vi "Bulk Example.vi"() -> ()   [LabVIEW 2010]
doc: "This VI shows how to use group reads and writes."
uses:
  Type Defs/Typed Name Set.ctl
  Type Defs/Data Types.ctl
  Type Defs/Group Data.ctl
  Type Defs/File Format.ctl
  Type Defs/Single Tag.ctl
  Type Defs/Tag Grouping set.ctl
  Read tags into grouped data.vi
  Write grouped data to tags.vi
  Read Index Set.vi
  DataTypes/Double_Read Index Set.vi
  DataTypes/Array of String_Read Index Set.vi
  DataTypes/Array of Boolean_Read Index Set.vi
  DataTypes/Array of Single_Read Index Set.vi
  DataTypes/Array of Double_Read Index Set.vi
  DataTypes/Array of I8_Read Index Set.vi
  DataTypes/Array of I16_Read Index Set.vi
  DataTypes/Array of I32_Read Index Set.vi
  DataTypes/Array of I64_Read Index Set.vi
  DataTypes/Array of U64_Read Index Set.vi
  DataTypes/Array of U32_Read Index Set.vi
  DataTypes/Array of U16_Read Index Set.vi
  DataTypes/Array of U8_Read Index Set.vi
  DataTypes/Boolean_Read Index Set.vi
  DataTypes/String_Read Index Set.vi
  DataTypes/U8_Read Index Set.vi
  DataTypes/U16_Read Index Set.vi
  DataTypes/U32_Read Index Set.vi
  DataTypes/U64_Read Index Set.vi
  DataTypes/I8_Read Index Set.vi
  DataTypes/I16_Read Index Set.vi
  DataTypes/I32_Read Index Set.vi
  DataTypes/I64_Read Index Set.vi
  DataTypes/Single_Read Index Set.vi
  Write Index Set.vi
  DataTypes/Double_Write Index Set.vi
  DataTypes/Array of String_Write Index Set.vi
  DataTypes/Array of Boolean_Write Index Set.vi
  DataTypes/Array of Single_Write Index Set.vi
  DataTypes/Array of Double_Write Index Set.vi
  DataTypes/Array of I8_Write Index Set.vi
  DataTypes/Array of I16_Write Index Set.vi
  DataTypes/Array of I32_Write Index Set.vi
  DataTypes/Array of I64_Write Index Set.vi
  DataTypes/Array of U64_Write Index Set.vi
  DataTypes/Array of U32_Write Index Set.vi
  DataTypes/Array of U16_Write Index Set.vi
  DataTypes/Array of U8_Write Index Set.vi
  DataTypes/Boolean_Write Index Set.vi
  DataTypes/String_Write Index Set.vi
  DataTypes/U8_Write Index Set.vi
  DataTypes/U16_Write Index Set.vi
  DataTypes/U32_Write Index Set.vi
  DataTypes/U64_Write Index Set.vi
  DataTypes/I8_Write Index Set.vi
  DataTypes/I16_Write Index Set.vi
  DataTypes/I32_Write Index Set.vi
  DataTypes/I64_Write Index Set.vi
  DataTypes/Single_Write Index Set.vi
  Form Single Group.vi
  FGVs/Group Memory.vi
  Memory Block.vi
  DataTypes/Double_Memory Block.vi
  DataTypes/Array of String_Memory Block.vi
  DataTypes/Array of Boolean_Memory Block.vi
  DataTypes/Array of Single_Memory Block.vi
  DataTypes/Array of Double_Memory Block.vi
  DataTypes/Array of I8_Memory Block.vi
  DataTypes/Array of I16_Memory Block.vi
  DataTypes/Array of I32_Memory Block.vi
  DataTypes/Array of I64_Memory Block.vi
  DataTypes/Array of U64_Memory Block.vi
  DataTypes/Array of U32_Memory Block.vi
  DataTypes/Array of U16_Memory Block.vi
  DataTypes/Array of U8_Memory Block.vi
  DataTypes/Boolean_Memory Block.vi
  DataTypes/String_Memory Block.vi
  DataTypes/U8_Memory Block.vi
  DataTypes/U16_Memory Block.vi
  DataTypes/U32_Memory Block.vi
  DataTypes/U64_Memory Block.vi
  DataTypes/I8_Memory Block.vi
  DataTypes/I16_Memory Block.vi
  DataTypes/I32_Memory Block.vi
  DataTypes/I64_Memory Block.vi
  DataTypes/Single_Memory Block.vi
  Current Value Table.lvlib
panel:
  out "Mission Critical Tags by Type":T1[](array[typedef])
  out "Expected Error":errorcluster
  out "Mission Critical Tags":string[](array[string]) caption="Tags Out"
  out "error out":errorcluster
  out "Tag 1":dbl
  out "Tag 2":dbl
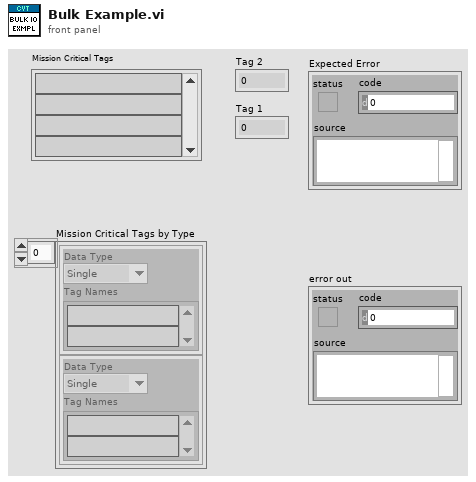
[diagram p1: front panel]
types:
  T1 = typedef "Current Value Table.lvlib/Typed Name Set.ctl" = cluster{"Data Type":T2, "Tag Names":string[]}
  T2 = typedef "Current Value Table.lvlib/Data Types.ctl" = enum16{"Double", "Single", "I64", "I32", "I16", "I8", "U64", "U32", "U16", "U8", "String", "Boolean", "Array of U8", "Array of U16", "Array of U32", "Array of U64", "Array of I64", "Array of I32", "Array of I16", "Array of I8", "Array of Double", "Array of Single", "Array of Boolean", "Array of String"}
  T3 = typedef "Current Value Table.lvlib/Group Data.ctl" = cluster{"Double":dbl[], "Single":sgl[], "I64":i64[], "I32":i32[], "I16":i16[], "I8":i8[], "U64":u64[], "U32":u32[], "U16":u16[], "U8":u8[], "String":string[], "Boolean":bool[], "Array of U8":cluster{"U8 Array":u8[]}[], "Array of U16":cluster{"U16 Array":u16[]}[], "Array of U32":cluster{"U32 Array":u32[]}[], "Array of U64":cluster{"U64 Array":u64[]}[], "Array of I64":cluster{"I64 Array":i64[]}[], "Array of I32":cluster{"I32 Array":i32[]}[], "Array of I16":cluster{"I16 Array":i16[]}[], "Array of I8":cluster{"I8 Array":i8[]}[], "Array of Double":cluster{"DBL Array":dbl[]}[], "Array of Single":cluster{"SGL Array":sgl[]}[], "Array of Boolean":cluster{"Boolean Array":bool[]}[], "Array of String":cluster{"String Array":string[]}[]}
  T4 = typedef "Current Value Table.lvlib/File Format.ctl" = cluster{"Tags":T5[], "Group Listings":T6[]}
  T5 = typedef "Current Value Table.lvlib/Single Tag.ctl" = cluster{"Data Type":T2, "Name":string, "Value":string, "Description":string}
  T6 = typedef "Current Value Table.lvlib/Tag Grouping set.ctl" = cluster{"Group":string, "Tag Names":string[]}
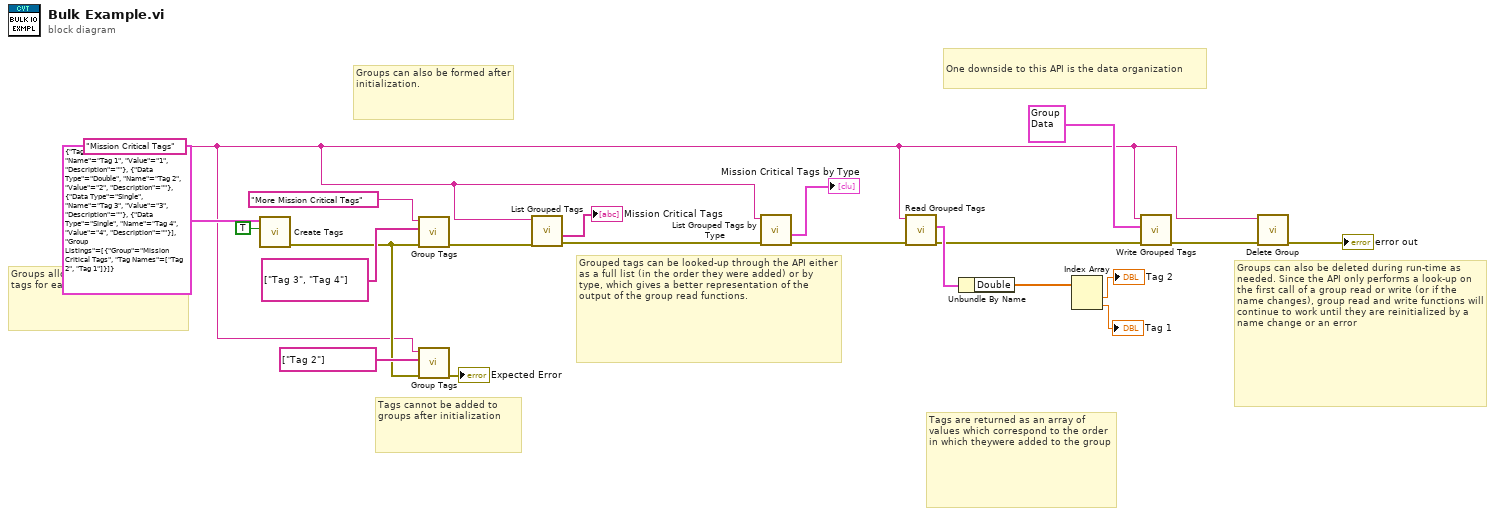
[diagram p0: block diagram]
diagram:
  w1 = "Mission Critical Tags" ("Group")
  # "Grouped tags can be looked-up through the API either as a full list (in the order they were added) or by type, which gives a better representation of the output of the group read functions."
  # "Groups can also be deleted during run-time as needed. Since the API only performs a look-up on the first call of a group read or write (or if the name changes), group read and write functions will continue to work until they are reinitialized by a name change or an error"
  # "Tags cannot be added to groups after initialization"
  # "One downside to this API is the data organization"
  # "Tags are returned as an array of  values which correspond to the order in which theywere added to the group"
  # "Groups can also be formed after initialization."
  # "Groups allow you to name a set of tags for easy access"
  n1 = call "Create Tags.vi"("Clear Table? (F)"=TRUE ("Clear Engine?"), "CVT Tags to Create"=T4 {"Tags"=[{"Data Type"=enum."Double", "Name"="Tag 1", "Value"="1", "Description"=""}, {"Data Type"=enum."Double", "Name"="Tag 2", "Value"="2", "Description"=""}, {"Data Type"=enum."Single", "Name"="Tag 3", "Value"="3", "Description"=""}, {"Data Type"=enum."Single", "Name"="Tag 4", "Value"="4", "Description"=""}], "Group Listings"=[{"Group"="Mission Critical Tags", "Tag Names"=["Tag 2", "Tag 1"]}]} ("CVT File Data")) -> ("error out"=w8:errorcluster)  [unwired: 9 in]
  n2 = call "Group Tags.vi"("error in (no error)"=w8, "Tag Names"=string[] ["Tag 3", "Tag 4"], "Group"="More Mission Critical Tags") -> ("error out"=w18:errorcluster)  [unwired: 8 in]
  n3 = call "Group Tags.vi"("error in (no error)"=w8, "Tag Names"=string[] ["Tag 2"], "Group"=w1) -> ("error out"=→"Expected Error":errorcluster)  [unwired: 8 in]
  n4 = call "List Grouped Tags.vi"("error in (no error)"=w18, "Group"=w1) -> ("error out"=w4:errorcluster, "Tags Out"=→"Mission Critical Tags":string[])  [unwired: 8 in]
  n5 = call "List Grouped Tags by Type.vi"("error in (no error)"=w4, "Group"=w1) -> ("error out"=w5:errorcluster, "Tags Out"=→"Mission Critical Tags by Type":T1[])  [unwired: 8 in]
  n6 = call "Read Grouped Tags.vi"("error in (no error)"=w5, "Group"=w1) -> ("error out"=w13:errorcluster, "Data"=w17:T3)  [unwired: 8 in]
  n7 = Unbundle By Name(w17) -> ("Double"=w16:dbl[])
  n8 = Index Array(array=w16) -> (element #1=→"Tag 2":dbl, element #2=→"Tag 1":dbl)  [unwired: 2 in]
  n9 = call "Write Grouped Tags.vi"("error in (no error)"=w13, "Data"=T3 {"Double"=[0.0, 0.0], "Single"=[], "I64"=[], "I32"=[], "I16"=[], "I8"=[], "U64"=[], "U32"=[], "U16"=[], "U8"=[], "String"=[], "Boolean"=[], "Array of U8"=[], "Array of U16"=[], "Array of U32"=[], "Array of U64"=[], "Array of I64"=[], "Array of I32"=[], "Array of I16"=[], "Array of I8"=[], "Array of Double"=[], "Array of Single"=[], "Array of Boolean"=[], "Array of String"=[]}, "Group"=w1) -> ("error out"=w7:errorcluster)  [unwired: 8 in]
  n10 = call "Delete Group.vi"("error in (no error)"=w7, "Group"=w1) -> ("error out"=→"error out":errorcluster)  [unwired: 9 in]
